vi "Update active by name.vi"(8 "error in (no error)":errorcluster, 9 "Active":bool, 10 "Name":string, 11 "Scheduile Array in":refnum<class "Scheduile Array.lvclass">) -> (0 "error out":errorcluster, 3 "Scheduile Array out":refnum<class "Scheduile Array.lvclass">)   [LabVIEW 2015, in "Scheduile Array.lvclass"]
uses:
  Scheduile Array.lvclass
  Schedule.lvclass
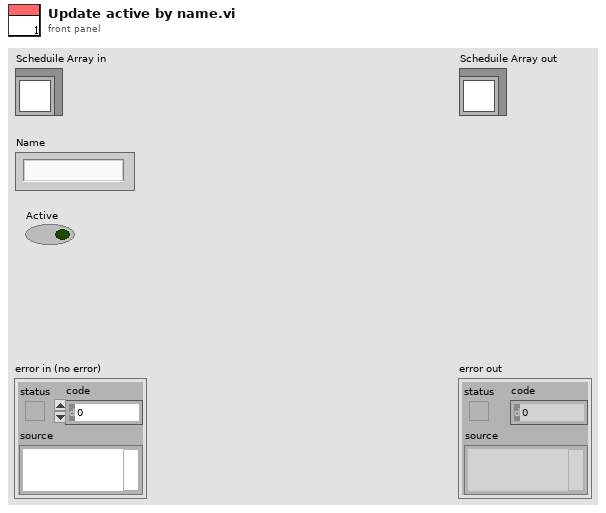
[diagram p1: front panel]
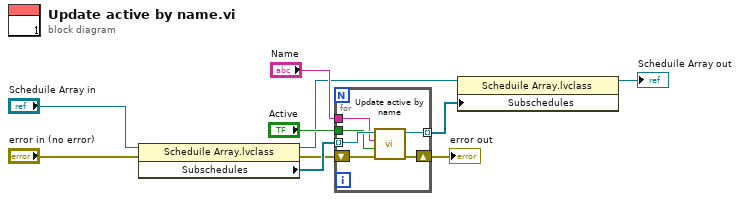
[diagram p0: block diagram]
diagram:
  n1 = property class="Scheduile Array.lvclass"(reference="Scheduile Array in", error in="error in (no error)") -> (reference out=w6:refnum<class "Scheduile Array.lvclass">, error out=w2:errorcluster, "Subschedules"=w9:refnum<class "Schedule.lvclass">[])
  n2 = for {
    tunnel: w9 -> [w16] mode=indexing
    tunnel: "Name" -> [w15]
    tunnel: "Active" -> [w14]
    shift-right: [w12] -> w1
    shift-left: w2 -> [w13]
    tunnel: [w11] -> w5 mode=indexing
    n3 = call-dynamic "Update active by name.vi"("error in (no error)"=w13, "Active"=w14, "Name"=w15, "Schedule in"=w16) -> ("error out"=w12:errorcluster, "Schedule out"=w11:refnum<class "Schedule.lvclass">)  [unwired: 6 in]
  }
  "error out" <- w1
  n4 = property class="Scheduile Array.lvclass"(reference=w6, "Subschedules"=w5) -> (reference out=→"Scheduile Array out":refnum<class "Scheduile Array.lvclass">)  [unwired: 1 in, 1 out]
